vi "FuncImg-Extract selected ROIs data-Core.vi"(9 "System Cluster":T7 {"ROI number" min=1 format="ROI %.0f"}, 10 "Input cluster":T3={"Channel A?"=FALSE, "Cycle length (us)"=0.0, "[Pixels in ROI]"=[], "Z-Stack Header data"={"Number of POI"=0, "Number of Miniscans"=0, "Number of Trials"=0, "Number of Cycles "=0, "# Averaged Frames"=0, "Laser power (%)"=0, "Pockels"=0.0, "Acquisition Length (sec)"=0.0, "Fill time (us)"=0.0, "DwellTime (us)"=0.0, "Miniscan Dwell time per pixel (us)"=0.0, "PMT 1"=0.0, "PMT 2"=0.0, "Back Apperture"=0.0, "Zoom"=0.0, "Number of Pixels in Miniscan"=0, "Frame Size"=200, "Field of View"=0.0, "X centre"=0.0, "Y centre"=0.0, "AOL Z"=0.0}, "[ROI Time (us)]"=[], "Path out"=path "", "Version index"=0} {"Z-Stack Header data"."Frame Size" items=["100X100"=100, "128X128"=128, "200X200"=200, "256X256"=256, "512X512"=512, "1024x1024"=1024, "2048x2048"=2048]; "Z-Stack Header data"."Back Apperture" format="%#.6g"; "Z-Stack Header data"."Pockels" format="%#.6g"; "Z-Stack Header data"."PMT 2" format="%#.6g"; "Z-Stack Header data"."PMT 1" format="%#.6g"; "Z-Stack Header data"."Miniscan Dwell time per pixel (us)" format="%#.6g"; "Z-Stack Header data"."Zoom" format="%#.6g"; "Z-Stack Header data"."DwellTime (us)" format="%#.6g"; "Z-Stack Header data"."Acquisition Length (sec)" format="%#.6g"; "Z-Stack Header data"."Fill time (us)" format="%#.6g"}) -> (0 "error IO":errorcluster, 1 "Points per trial":i32, 3 "Interface-Data format definition":T4)   [LabVIEW 2017]
uses:
  xcontrol/Interface VIs/Interface typedefs/Interface-ROI selection cluster.ctl
  Typedefs/ROI ID Enum.ctl
  xcontrol/Interface VIs/Interface typedefs/Interface-Data format definition.ctl
  xcontrol/Typedefs/Xctl-XY data type definition.ctl
  xcontrol/Typedefs/Xctrl-ROI type enum.ctl
  Experiment header interface/Typedefs/Header parameters cluster-Zstack.ctl
  Typedefs/Frame Size.ctl
  xcontrol/XGrapher.xctl
panel:
  # "<--- Timeline data already decimated\n          for memory efficiency."
  # "Zstack header parameters"
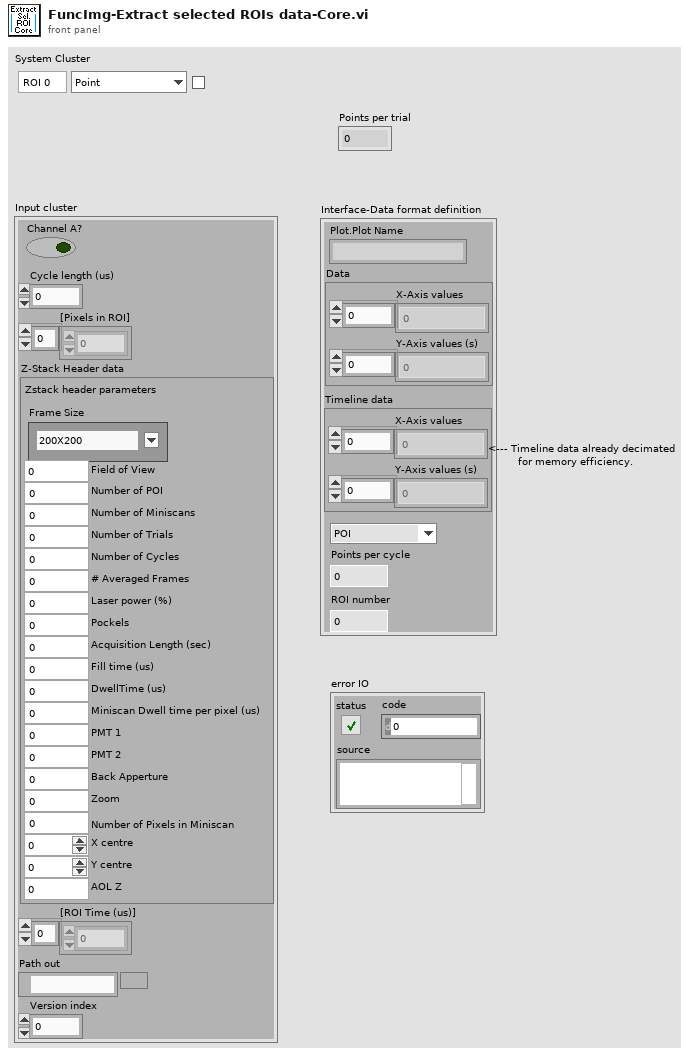
[diagram p1: front panel]
types:
  T1 = typedef "Header parameters cluster-Zstack.ctl" = cluster{"Number of POI":u16, "Number of Miniscans":u16, "Number of Trials":u16, "Number of Cycles ":u16, "# Averaged Frames":u16, "Laser power (%)":u8, "Pockels":dbl, "Acquisition Length (sec)":dbl, "Fill time (us)":dbl, "DwellTime (us)":dbl, "Miniscan Dwell time per pixel (us)":dbl, "PMT 1":dbl, "PMT 2":dbl, "Back Apperture":dbl, "Zoom":dbl, "Number of Pixels in Miniscan":u16, "Frame Size":T2, "Field of View":dbl, "X centre":dbl, "Y centre":dbl, "AOL Z":dbl}
  T2 = typedef "Frame Size.ctl" = u16
  T3 = cluster{"Channel A?":bool, "Cycle length (us)":dbl, "[Pixels in ROI]":i32[], "Z-Stack Header data":T1, "[ROI Time (us)]":dbl[], "Path out":path, "Version index":i32}
  T4 = typedef "Interface-Data format definition.ctl" = cluster{"Plot.Plot Name":string, "Data":T5, "Timeline data":T5, "Type":T6, "Points per cycle":u16, "ROI number":u16}
  T5 = typedef "XGrapher.xctl/Xctl-XY data type definition.ctl" = cluster{"X-Axis values":sgl[], "Y-Axis values (s)":sgl[]}
  T6 = typedef "Xctrl-ROI type enum.ctl" = enum16{"POI", "Mini-scan", "Group"}
  T7 = typedef "Interface-ROI selection cluster.ctl" = cluster{"ROI number":i32, "ROI ID":T8, "Visibility":bool}
  T8 = typedef "ROI ID Enum.ctl" = enum16{"Point", "MiniScan", "Comp. MiniScan", "Rectangle", "Comp. volume", "Arb. plane point", "None"}
  T9 = typedef "Interface-ROI type enum.ctl" = enum16{"POI", "Mini-scan"}
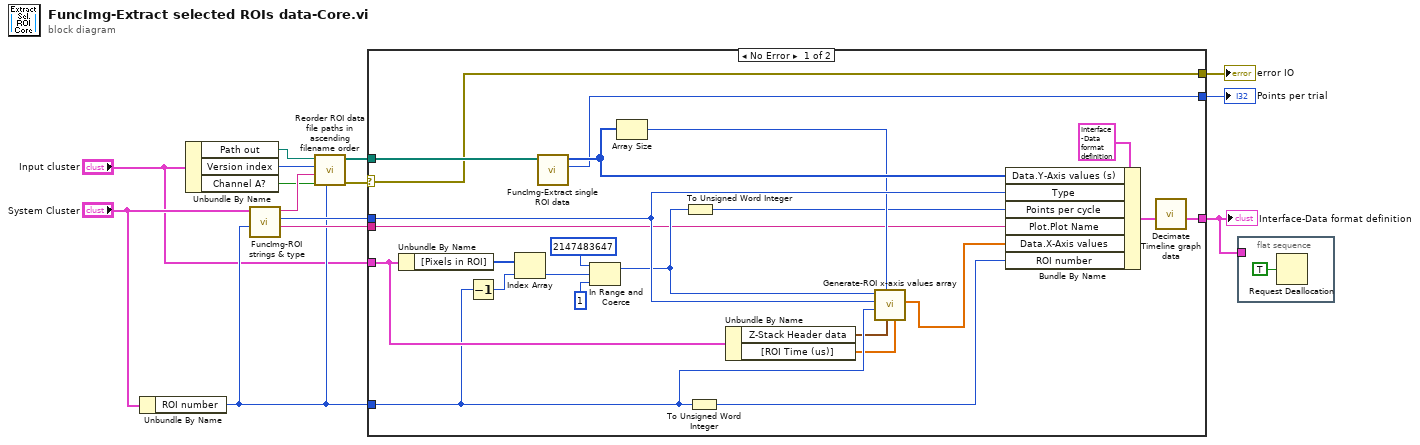
[diagram p0: block diagram]
diagram:
  n1 = Unbundle By Name("System Cluster") -> ("ROI number"=w6:i32)
  n2 = Unbundle By Name("Input cluster") -> ("Path out"=w13:path, "Version index"=w14:i32, "Channel A?"=w10:bool)
  n3 = call "FuncImg-ROI strings & type.vi"("ROI number"=w6, "ROI visibility cluster"="System Cluster") -> ("Plot name"=w9:string, "ROI type"=w12:T9, "ROI ID string"=w11:string)  [unwired: 7 in]
  n4 = call "Reorder ROI data file paths in ascending filename order.vi"("ROI number"=w6, "Channel A?"=w10, "ROI ID string"=w11, "ROI file format version"=w14, "Dataset directory path"=w13) -> ("Error out"=w4:errorcluster, "Reordered file paths in ascending file-name order"=w2:path[])  [unwired: 5 in]
  n5 = case shown="No Error" w4 {
    selector: w4 -> [w19 w38]
    tunnel: w12 -> [w36 _]
    tunnel: w2 -> [w34 _]
    tunnel: w9 -> [w24 _]
    tunnel: [w23 _] -> w8
    tunnel: w6 -> [w17 _]
    tunnel: "Input cluster" -> [w18 _]
    tunnel: [w20 _] -> w1
    tunnel: [w19 w38] -> w3
    frame No Error {
      n6 = Unbundle By Name(w18) -> ("[Pixels in ROI]"=w37:i32[])
      n7 = Decrement(x=w17) -> (x-1=w31:i32)
      n8 = Index Array(array=w37, index=w31) -> (element=w25:i32)
      n9 = call "FuncImg-Extract single ROI data.vi"("Reordered file paths in ascending file-name order"=w34) -> ("Points per trial"=w23:i32, "Data. Y-Axis values"=w35:i32[])  [unwired: 9 in]
      n10 = In Range and Coerce(upper limit=2147483647, x=w25, lower limit=1) -> (coerced(x)=w29:i32)  [unwired: 1 out]
      n11 = Array Size(array=w35) -> (size(s)=w32:i32)
      n12 = To Unsigned Word Integer(number=w29) -> (unsigned 16bit integer=w28:u16)
      n13 = To Unsigned Word Integer(number=w17) -> (unsigned 16bit integer=w30:u16)
      n14 = Unbundle By Name(w18) -> ("Z-Stack Header data"=w16:T1, "[ROI Time (us)]"=w15:dbl[])
      n15 = call "Generate-ROI x-axis values array.vi"("[ROI Time(us)]"=w15, "Header data"=w16, "Number of points in Y-axis array"=w32, "ROI number"=w17, "Type"=w36, "Pixels in ROI"=w29) -> ("ROI X-axis values array (sec)"=w22:sgl[])  [unwired: 5 in]
      n16 = Bundle By Name(cluster=T4 {"Plot.Plot Name"="", "Data"={"X-Axis values"=[], "Y-Axis values (s)"=[]}, "Timeline data"={"X-Axis values"=[], "Y-Axis values (s)"=[]}, "Type"=enum."POI", "Points per cycle"=0, "ROI number"=0}, "Data.Y-Axis values (s)"=w35, "Type"=w36, "Points per cycle"=w28, "Plot.Plot Name"=w24, "Data.X-Axis values"=w22, "ROI number"=w30) -> (w21:T4)
      n17 = call "Decimate Timeline graph data.vi"("Data in"=w21) -> ("Data out"=w20:T4)  [unwired: 10 in]
    }
    frame Error {
    }
  }
  "Interface-Data format definition" <- w1
  "Points per trial" <- w8
  "error IO" <- w3
  n18 = flat-sequence {
    tunnel: w1 -> [_]
    frame #0 {
      n19 = Request Deallocation(TRUE ("flag")) -> ()
    }
  }
